vi "rteta.v1.3.vi"() -> ()   [LabVIEW 2016]
uses:
  xcontrol/Start Button.xctl
  <vilib>/silver_ctls/ArrayMatrixCluster/Real Matrix NI_Silver.ctl
  <vilib>/Instr/_visa.llb/VISA Configure Serial Port (Instr).vi
  <instrlib>/Tektronix TDS 200 1000 2000 Series/Public/Data/Read (Single Waveform).vi
  <vilib>/measure/maspectr.llb/FFT Spectrum (Mag-Phase) for 1 Chan.vi
  <vilib>/measure/maspectr.llb/FFT Spectrum (Real-Im) for 1 Chan.vi
  <instrlib>/Tektronix TDS 200 1000 2000 Series/Tektronix TDS 200 1000 2000 Series.lvlib
  <vilib>/measure/NI_MAPro.lvlib
panel:
  out "Real Matrix":T1
  out "Out Com":string="x"
  out "İlk Ayar":bool=TRUE
  out "phase":cluster{"f0":dbl, "df":dbl, "phase":dbl[]} {"phase" format="%.2p"; "f0" format="%0.2p"; "df" format="%0.2p"}
  out "magnitude":cluster{"f0":dbl, "df":dbl, "magnitude":dbl[]} {"magnitude" format="%.2p"; "f0" format="%0.2p"; "df" format="%0.2p"}
  out "imaginary part":T2 {"imaginary part" format="%.2p"; "f0" format="%0.2p"; "df" format="%0.2p"}
  out "real part":cluster{"f0":dbl, "df":dbl, "real part":dbl[]} {"real part" format="%.2p"; "f0" format="%0.2p"; "df" format="%0.2p"}
  out "Waveform Data":waveform(dbl)(graph)
  in  "Osiloskop Portu":refnum<visa-resource-name>="COM1"
  in  "Start Button":dbl(xcontrol)
  in  "Frekans (kHz)":i32(slide)=1 caption="Amplitude(V)" scale=0.0..100.0
  in  "Reset Dafault":bool
  in  "Teta":i32(slide) scale=0.0..360.0
  in  "Sinyal Jeneratörü Portu":refnum<visa-resource-name>="COM4"
  in  "OUTPUT":bool=TRUE caption="Output"
  in  "Offset":i32(slide) scale=0.0..10.0
  in  "Amplitude(V)":i32(slide)=5 scale=0.0..20.0
  in  "cmdOrjin":bool
  in  "cmdStop":bool
  in  "Motor Sürücü Portu":refnum<visa-resource-name>="COM3"
  # "Frekans"
  # "Teta"
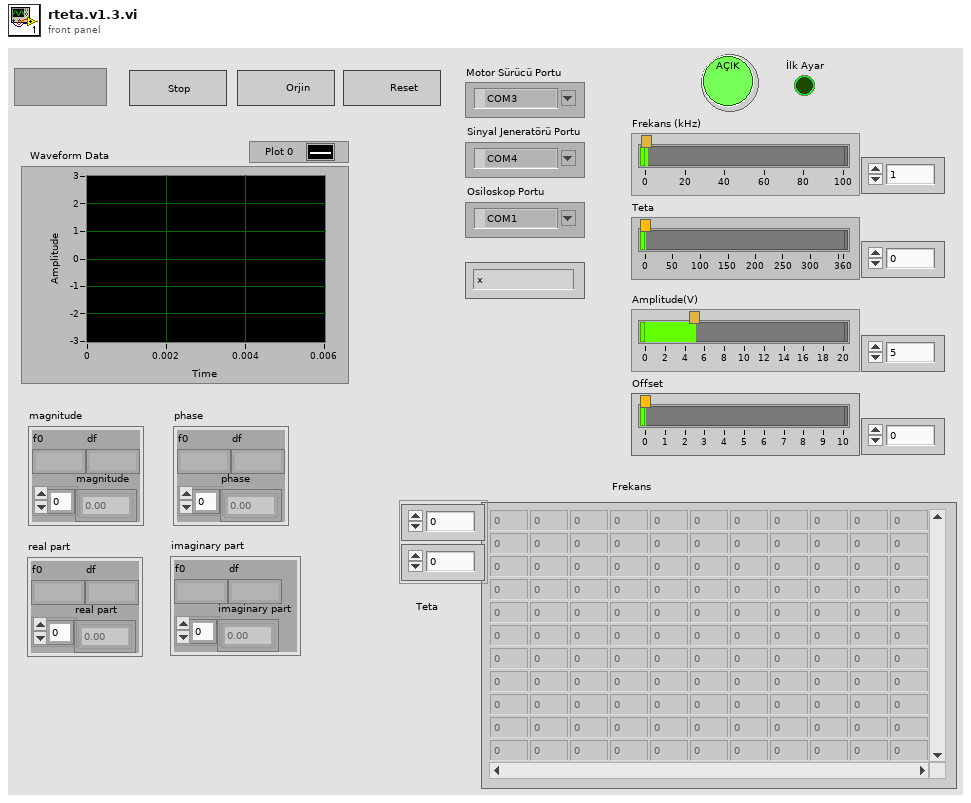
[diagram p1: front panel]
types:
  T1 = typedef "Real Matrix NI_Silver.ctl" = dbl[][]
  T2 = cluster{"f0":dbl, "df":dbl, "imaginary part":dbl[]}
  T3 = cluster{"Baud Rate":u32, "Parity":u16, "Stop Bits":u16, "Flow Control":u16}
  T4 = typedef "NI_Matrix.lvlib/RealMatrix.ctl" = dbl[][]
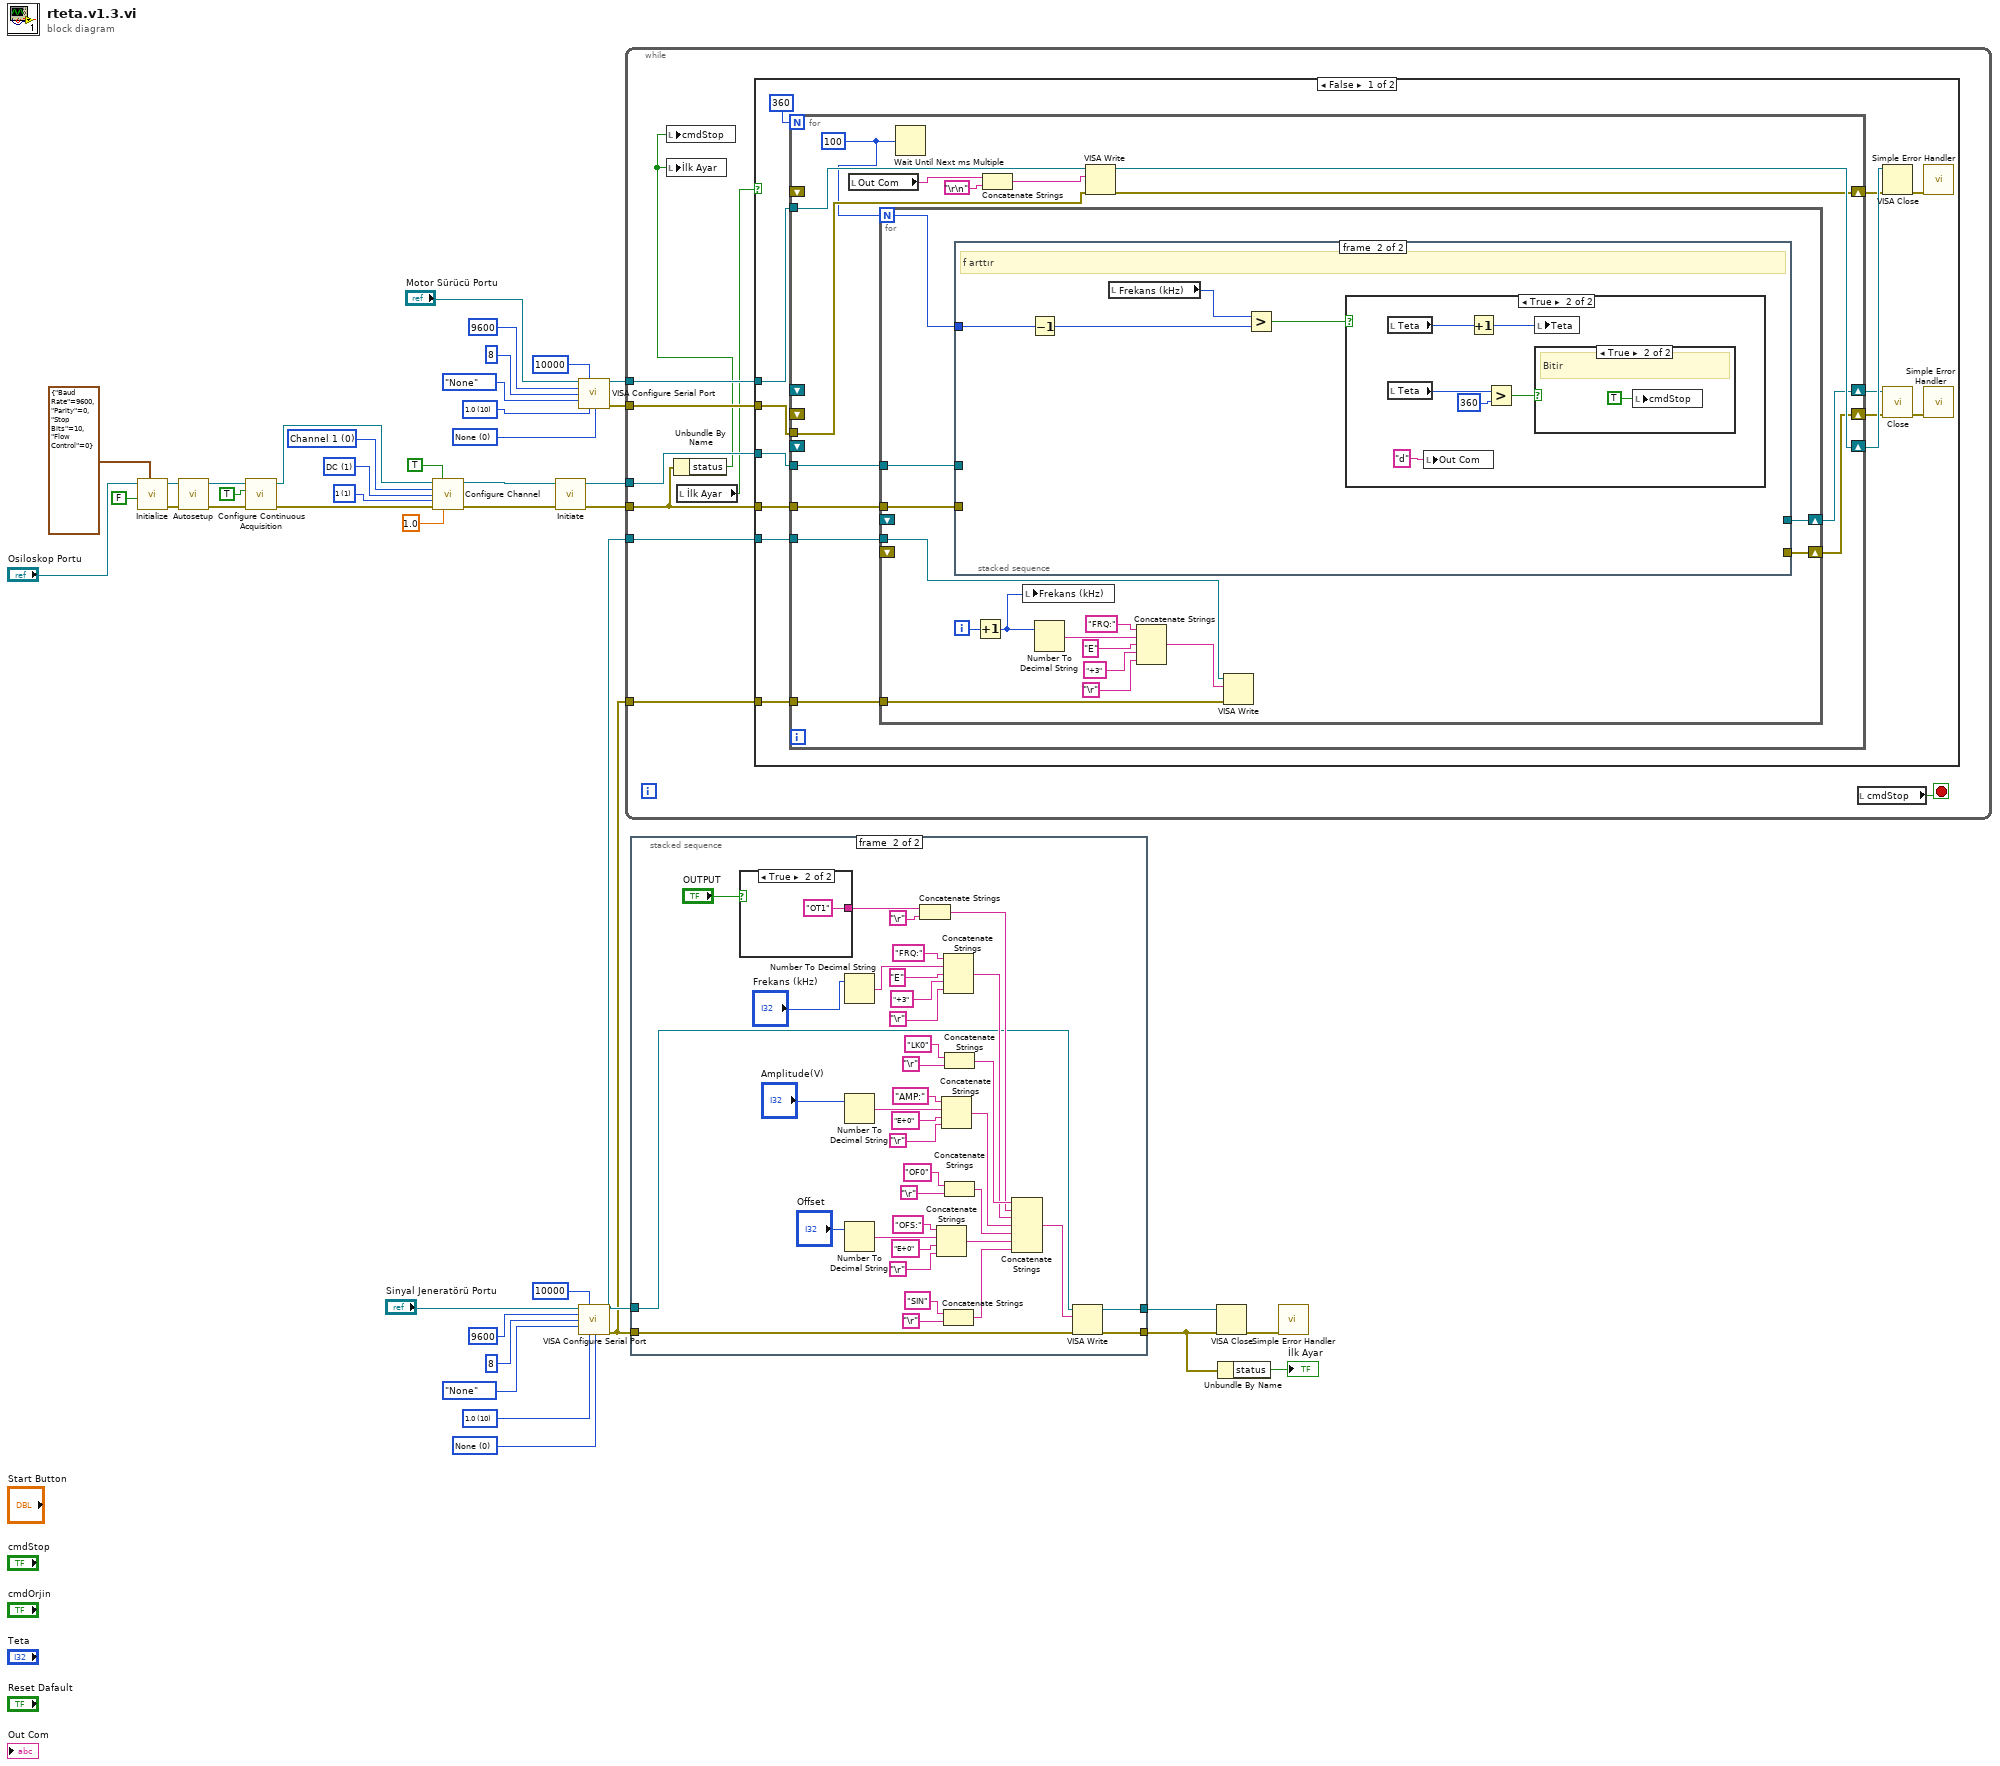
[diagram p0: block diagram]
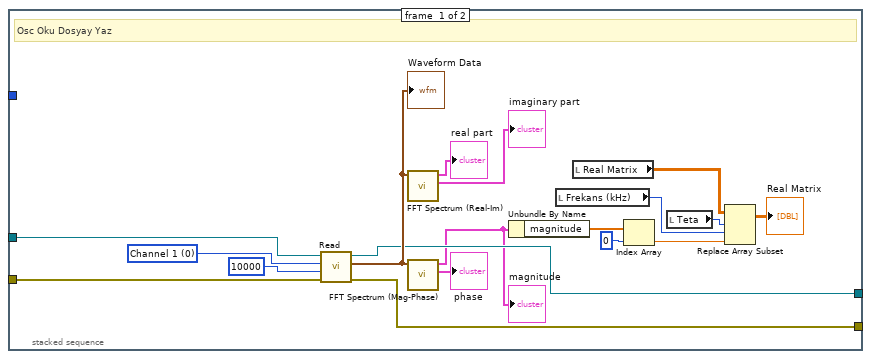
[diagram p2: hidden frame]
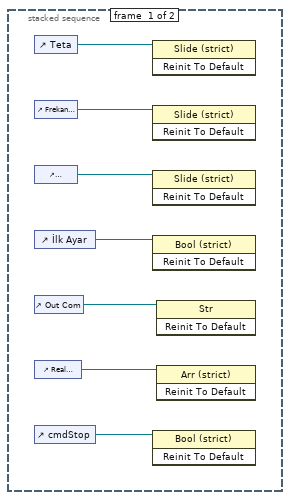
[diagram p6: hidden frame]
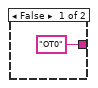
[diagram p7: hidden frame]
diagram:
  w10 = 1 items=["AC", "DC", "Ground"] ("Vertical Coupling (1: DC)")
  w11 = 0 items=["Channel 1", "Channel 2", "Channel 3", "Channel 4", "Math", "Reference A", "Reference B", "Reference C", "Reference D"] ("Channel (0: Channel 1)")
  w13 = 1 items=["1"=1, "10"=10, "20"=20, "50"=50, "100"=100, "500"=500, "1000"=1000] ("Probe Attenuation (10: 10X)")
  w34 = u16 0 items=["None", "XON/XOFF", "RTS/CTS", "XON/XOFF & RTS/CTS", "DTR/DSR", "XON/XOFF & DTR/DSR"] ("flow control (0:none)")
  w33 = u16 10 items=["1.0"=10, "1.5"=15, "2.0"=20] ("stop bits (10: 1 bit)")
  w35 = u16 0 items=["None", "XON/XOFF", "RTS/CTS", "XON/XOFF & RTS/CTS", "DTR/DSR", "XON/XOFF & DTR/DSR"] ("flow control (0:none)")
  w36 = u16 10 items=["1.0"=10, "1.5"=15, "2.0"=20] ("stop bits (10: 1 bit)")
  n1 = call <instrlib>:"Initialize.vi"("Serial Configuration"=T3 {"Baud Rate"=9600, "Parity"=0, "Stop Bits"=10, "Flow Control"=0} ("Osiloskop Config"), "Reset? (T: Yes)"=FALSE, "VISA resource name"="Osiloskop Portu") -> ("error out"=w23:errorcluster, "VISA resource name out"=w24:refnum<visa-resource-name>)  [unwired: 2 in, 5 out]
  n2 = call <instrlib>:"Autosetup.vi"("error in (no error)"=w23, "VISA resource name"=w24) -> ("error out"=w25:errorcluster, "VISA resource name out"=w26:refnum<visa-resource-name>)  [unwired: 8 out]
  n3 = call <instrlib>:"Configure Continuous Acquisition.vi"("error in (no error)"=w25, "Enable Continuous Acquisition Mode (True)"=TRUE, "VISA resource name"=w26) -> ("error out"=w14:errorcluster, "VISA resource name out"=w17:refnum<visa-resource-name>)  [unwired: 7 out]
  n4 = call <instrlib>:"Configure Channel.vi"("VISA resource name"=w17, "Enable Channel (True)"=TRUE, "Channel (0: Channel 1)"=w11, "Vertical Coupling (1: DC)"=w10, "Probe Attenuation (10: 10X)"=w13, "error in (no error)"=w14, "Vertical Range (10.0 V/div)"=1.0) -> ("VISA resource name out"=w16:refnum<visa-resource-name>, "error out"=w15:errorcluster)  [unwired: 7 in]
  n5 = call <instrlib>:"Initiate.vi"("error in (no error)"=w15, "VISA resource name"=w16) -> ("error out"=w19:errorcluster, "VISA resource name out"=w20:refnum<visa-resource-name>)  [unwired: 8 out]
  n6 = call-poly "VISA Configure Serial Port"("VISA resource name"="Motor Sürücü Portu", "timeout (10sec)"=u32 10000, "baud rate (9600)"=u32 9600, "data bits (8)"=u16 8, "parity (0:none)"=enum16{"None", "Odd", "Even", "Mark", "Space"}."None", "stop bits (10: 1 bit)"=w36, "flow control (0:none)"=w35) -> ("VISA resource name out"=w18:refnum<visa-resource-name>, "error out"=w4:errorcluster)  [unwired: 7 in]
  n7 = call-poly "VISA Configure Serial Port"("VISA resource name"="Sinyal Jeneratörü Portu", "timeout (10sec)"=u32 10000, "baud rate (9600)"=u32 9600, "data bits (8)"=u16 8, "parity (0:none)"=enum16{"None", "Odd", "Even", "Mark", "Space"}."None", "stop bits (10: 1 bit)"=w33, "flow control (0:none)"=w34) -> ("VISA resource name out"=w7:refnum<visa-resource-name>, "error out"=w6:errorcluster)  [unwired: 7 in]
  n8 = while {
    tunnel: w20 -> [w50]
    tunnel: w19 -> [w43]
    tunnel: w18 -> [w49]
    tunnel: w7 -> [w48]
    tunnel: w6 -> [w47]
    tunnel: w4 -> [w46]
    stop <- w45 stop-if-true
    n9 = Unbundle By Name(w43) -> ("status"=w42:bool)
    n10 = local write "cmdStop"(w42) -> ()
    n11 = local write "İlk Ayar"(w42) -> ()
    n12 = local read "İlk Ayar"() -> (w44:bool)
    n13 = case shown="False" w44 {
      tunnel: w50 -> [w63 _]
      tunnel: w43 -> [w62 _]
      tunnel: w49 -> [w61 _]
      tunnel: w46 -> [w60 _]
      tunnel: w48 -> [w58 _]
      tunnel: w47 -> [w57 _]
      frame False {
        n14 = for {
          N: 360 -> [_]
          tunnel: w63 -> [w76]
          tunnel: w62 -> [w77]
          tunnel: w61 -> [w71]
          tunnel: w60 -> [w70]
          tunnel: w58 -> [w75]
          tunnel: w57 -> [w74]
          shift-right: [w69] -> w55
          shift-left: _ -> [_]
          shift-right: [w68] -> w54
          shift-left: _ -> [_]
          shift-right: [w66] -> w52
          shift-left: _ -> [_]
          shift-right: [w65] -> w51
          shift-left: _ -> [_]
          w64 = u32 100 ("millisecond multiple")
          n15 = local read "Out Com"() -> (w67:string)
          n16 = for {
            N: w64 -> [w80]
            tunnel: w76 -> [w92]
            tunnel: w77 -> [w91]
            tunnel: w75 -> [w88]
            tunnel: w74 -> [w89]
            shift-right: [w79] -> w66
            shift-left: _ -> [_]
            shift-right: [w78] -> w65
            shift-left: _ -> [_]
            i -> [w90]
            n17 = stacked-sequence {
              tunnel: w92 -> [w104 _]
              tunnel: w91 -> [w103 _]
              tunnel: w80 -> [_ w112]
              tunnel: [w102 _] -> w79
              tunnel: [w101 _] -> w78
              frame #0 {
                w109 = u16 0 items=["Channel 1", "Channel 2", "Channel 3", "Channel 4", "Math", "Reference A", "Reference B", "Reference C", "Reference D"] ("Channel B (1: Channel 2)")
                # "Osc Oku Dosyay Yaz"
                n18 = call-poly <instrlib>:"Read.vi"("error in (no error)"=w103, "Timeout (10000 ms)"=u32 10000 ("Timeout (10000 ms) 2"), "Source (0: Channel 1)"=w109, "VISA resource name"=w104) -> ("error out"=w102:errorcluster, "Waveform Data"=w105:waveform(dbl), "VISA resource name out"=w101:refnum<visa-resource-name>)  [unwired: 5 out]
                "Waveform Data" <- w105
                n19 = call-poly <vilib>:"FFT Spectrum (Real-Im).vi"("time signal"=w105) -> ("imaginary part"=→"imaginary part":T2, "real part"=→"real part":cluster{"f0":dbl, "df":dbl, "real part":dbl[]})  [unwired: 6 in, 3 out]
                n20 = call-poly <vilib>:"FFT Spectrum (Mag-Phase).vi"("time signal"=w105) -> ("phase"=→"phase":cluster{"f0":dbl, "df":dbl, "phase":dbl[]}, "magnitude"=w100:cluster{"f0":dbl, "df":dbl, "magnitude":dbl[]})  [unwired: 6 in, 3 out]
                "magnitude" <- w100
                n21 = Unbundle By Name(w100) -> ("magnitude"=w97:dbl[])
                n22 = local read "Frekans (kHz)"() -> (w94:i32)
                n23 = local read "Real Matrix"() -> (w98:T1)
                n24 = Index Array(array=w97, index=0) -> (element=w95:dbl)
                n25 = local read "Teta"() -> (w93:i32)
                n26 = Replace Array Subset ("Set Matrix Elements")(array=w98, new element=w95, index (row)=w93, index (col)=w94) -> (→"Real Matrix":T4)
              }
              frame #1 {
                # "f arttır"
                n27 = Decrement(x=w112) -> (x-1=w111:i32)
                n28 = local read "Frekans (kHz)"() -> (w113:i32)
                n29 = Greater?(x=w113, y=w111) -> (0:w114:bool)
                n30 = case shown="True" w114 {
                  frame False {
                  }
                  frame True {
                    n31 = local read "Teta"() -> (w116:i32)
                    n32 = local read "Teta"() -> (w118:i32)
                    n33 = local write "Out Com"("d" ("Out Com")) -> ()
                    n34 = Increment(x=w116) -> (x+1=w117:i32)
                    n35 = Greater?(x=w118, y=360) -> (0:w120:bool)
                    n36 = local write "Teta"(w117) -> ()
                    n37 = case shown="True" w120 {
                      frame False {
                      }
                      frame True {
                        # "Bitir"
                        n38 = local write "cmdStop"(TRUE ("cmdStop")) -> ()
                      }
                    }
                  }
                }
              }
            }
            n39 = Increment(x=w90) -> (x+1=w81:i32)
            n40 = local write "Frekans (kHz)"(w81) -> ()
            n41 = Number To Decimal String(number=w81) -> (decimal integer string=w85:string)  [unwired: 1 in]
            n42 = Concatenate Strings("FRQ:", w85, "E", "+3", "\r") -> (w82:string)
            n43 = VISA Write(VISA resource name=w88, write buffer=w82, error in (no error)=w89) -> ()  [unwired: 3 out]
          }
          n44 = Wait Until Next ms Multiple(millisecond multiple=w64) -> ()  [unwired: 1 out]
          n45 = Concatenate Strings(w67, "\r\n") -> (w72:string)
          n46 = VISA Write(VISA resource name=w71, write buffer=w72, error in (no error)=w70) -> (VISA resource name out=w69:refnum<visa-resource-name>, error out=w68:errorcluster)  [unwired: 1 out]
        }
        n47 = VISA Close(VISA resource name=w55, error in (no error)=w54) -> (error out=w56:errorcluster)
        n48 = call <instrlib>:"Close.vi"("error in (no error)"=w52, "VISA resource name"=w51) -> ("error out"=w53:errorcluster)  [unwired: 9 in]
        n49 = call <vilib>:"Simple Error Handler.vi"("error in (no error)"=w56) -> ()  [unwired: 4 in, 5 out]
        n50 = call <vilib>:"Simple Error Handler.vi"("error in (no error)"=w53) -> ()  [unwired: 4 in, 5 out]
      }
      frame True {
      }
    }
    n51 = local read "cmdStop"() -> (w45:bool)
  }
  n52 = stacked-sequence {
    tunnel: w7 -> [_ w132]
    tunnel: w6 -> [_ w131]
    tunnel: [_ w130] -> w5
    tunnel: [_ w129] -> w1
    frame #0 {
      n53 = control-ref of="Teta"() -> (w126:refnum<vi>)
      n54 = control-ref of="Frekans (kHz)"() -> (w128:refnum<vi>)
      n55 = control-ref of="Amplitude(V)"() -> (w127:refnum<vi>)
      n56 = control-ref of="İlk Ayar"() -> (w125:refnum<vi>)
      n57 = control-ref of="Out Com"() -> (w124:refnum<vi>)
      n58 = control-ref of="Real Matrix"() -> (w123:refnum<vi>)
      n59 = control-ref of="cmdStop"() -> (w122:refnum<vi>)
      n60 = invoke class="Slide (strict)" method="Reinit To Default"(reference=w126) -> ()  [unwired: 2 in, 3 out]
      n61 = invoke class="Slide (strict)" method="Reinit To Default"(reference=w128) -> ()  [unwired: 2 in, 3 out]
      n62 = invoke class="Slide (strict)" method="Reinit To Default"(reference=w127) -> ()  [unwired: 2 in, 3 out]
      n63 = invoke class="Bool (strict)" method="Reinit To Default"(reference=w125) -> ()  [unwired: 2 in, 3 out]
      n64 = invoke class="Bool (strict)" method="Reinit To Default"(reference=w122) -> ()  [unwired: 2 in, 3 out]
      n65 = invoke class="Str" method="Reinit To Default"(reference=w124) -> ()  [unwired: 2 in, 3 out]
      n66 = invoke class="Arr (strict)" method="Reinit To Default"(reference=w123) -> ()  [unwired: 2 in, 3 out]
    }
    frame #1 {
      n67 = case shown="True" "OUTPUT" {
        tunnel: ["OT0" "OT1"] -> w159
        frame False {
        }
        frame True {
        }
      }
      n68 = Number To Decimal String(number="Frekans (kHz)") -> (decimal integer string=w154:string)  [unwired: 1 in]
      n69 = Number To Decimal String(number="Amplitude(V)") -> (decimal integer string=w148:string)  [unwired: 1 in]
      n70 = Number To Decimal String(number="Offset") -> (decimal integer string=w141:string)  [unwired: 1 in]
      n71 = Concatenate Strings(w159, "\r") -> (w156:string)
      n72 = Concatenate Strings("OFS:", w141, "E+0", "\r") -> (w140:string)
      n73 = Concatenate Strings("AMP:", w148, "E+0", "\r") -> (w147:string)
      n74 = Concatenate Strings("FRQ:", w154, "E", "+3", "\r") -> (w153:string)
      n75 = Concatenate Strings("SIN", "\r") -> (w139:string)
      n76 = Concatenate Strings("LK0", "\r") -> (w157:string)
      n77 = Concatenate Strings("OF0", "\r") -> (w144:string)
      n78 = Concatenate Strings(w157, w156, w153, w147, w144, w140, w139) -> (w133:string)
      n79 = VISA Write(VISA resource name=w132, write buffer=w133, error in (no error)=w131) -> (VISA resource name out=w130:refnum<visa-resource-name>, error out=w129:errorcluster)  [unwired: 1 out]
    }
  }
  n80 = VISA Close(VISA resource name=w5, error in (no error)=w1) -> (error out=w3:errorcluster)
  n81 = Unbundle By Name(w1) -> ("status"=→"İlk Ayar":bool)
  n82 = call <vilib>:"Simple Error Handler.vi"("error in (no error)"=w3) -> ()  [unwired: 4 in, 5 out]
